vi "GetType.vi"(8 "error in (no error)":errorcluster, 11 "Configure Output Enable Msg":refnum<class "Configure Output Enable Msg.lvclass">) -> (0 "error out":errorcluster, 2 "Data Sample":variant, 3 "Configure Output Enable Msg":refnum<class "Configure Output Enable Msg.lvclass">)   [LabVIEW 2016, in "CS++Fgen.lvlib" / "Configure Output Enable Msg.lvclass"]
doc: "This VI delivers a sample of the data type format the message expects."
uses:
  Configure Output Enable Msg.lvclass
  Configure Output Enable Msg.lvclass/Configure Output Enable Msg.ctl
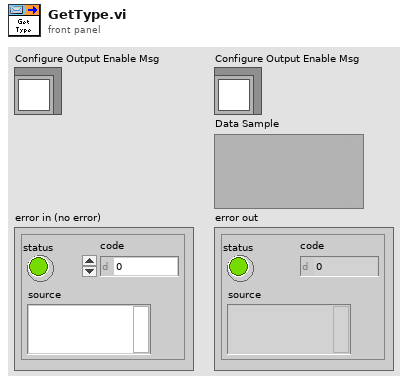
[diagram p1: front panel]
types:
  T1 = cluster{"channel name (\"CHANNEL1\")":string, "channel enabled (True)":bool}
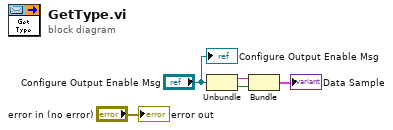
[diagram p0: block diagram]
diagram:
  n1 = Unbundle("Configure Output Enable Msg") -> (w2:string, w1:bool)
  n2 = Bundle("channel name (\"CHANNEL1\")"=w2, "channel enabled (True)"=w1) -> (→"Data Sample":T1)  [unwired: 1 in]
  "error out" <- "error in (no error)"
  "Configure Output Enable Msg" <- "Configure Output Enable Msg"
